vi "Read type.vi"(8 "error in (no error)":errorcluster, 11 "id in":refnum<class "id.lvclass">) -> (0 "error out":errorcluster, 2 "type":enum16{"none", "String", "Number", "NULL"}(ring), 3 "id out":refnum<class "id.lvclass">)   [LabVIEW 2015]
uses:
  id.lvclass
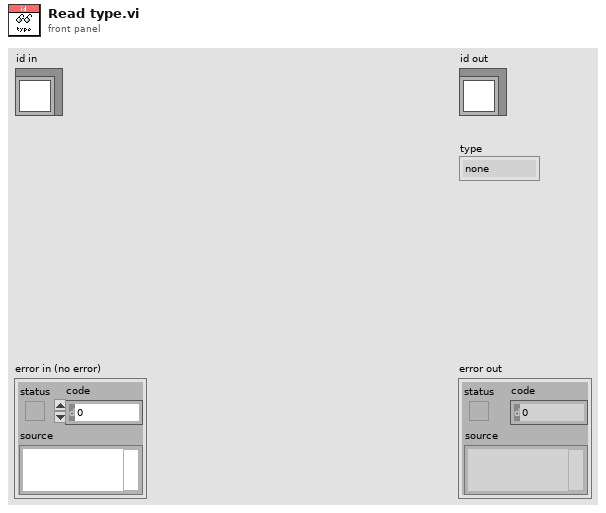
[diagram p1: front panel]
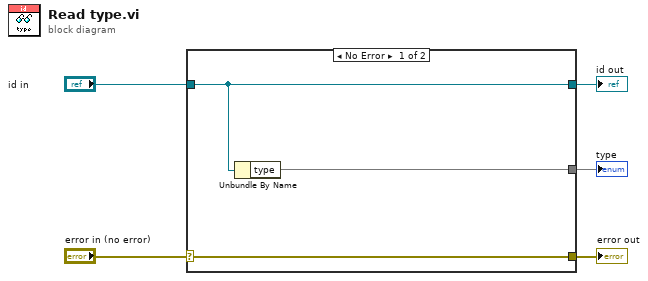
[diagram p0: block diagram]
diagram:
  n1 = case shown="No Error" "error in (no error)" {
    selector: "error in (no error)" -> [w8 w9]
    tunnel: [w8 w9] -> w4
    tunnel: [w7 w10] -> w2
    tunnel: "id in" -> [w7 w10]
    tunnel: [w6 _] -> w1
    frame No Error {
      n2 = Unbundle By Name(w7) -> ("type"=w6)
    }
    frame Error {
    }
  }
  "error out" <- w4
  "id out" <- w2
  "type" <- w1
